vi "compress to 8 bit imaq cast.vi"(8 "error in (no error)":errorcluster, 9 "Image Dst Out":T1, 10 "Bit depth":string, 11 "Refnum in":T1) -> (0 "error out":errorcluster, 3 "Refnum out":T1)   [LabVIEW 2020]
uses:
  IMAQ Image.ctl
  NI_Vision_Development_Module.lvlib
panel:
  in  "lose lowest bits":bool
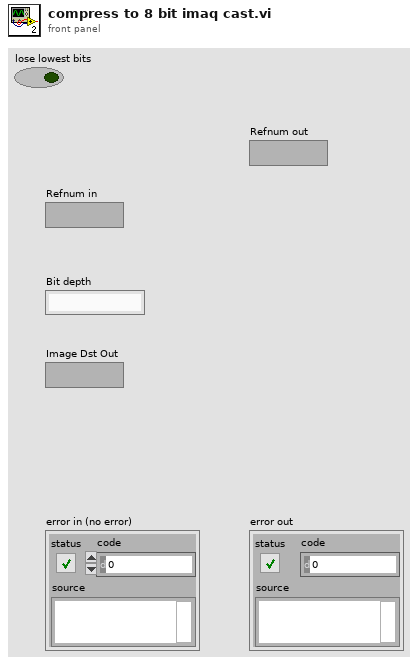
[diagram p1: front panel]
types:
  T1 = typedef "IMAQ Image.ctl" = refnum<image>
  T2 = typedef "Image Type" = u32
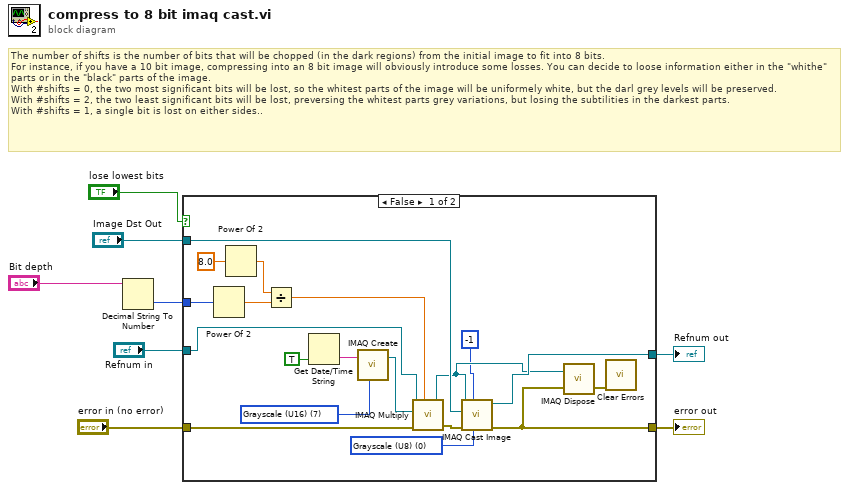
[diagram p0: block diagram]
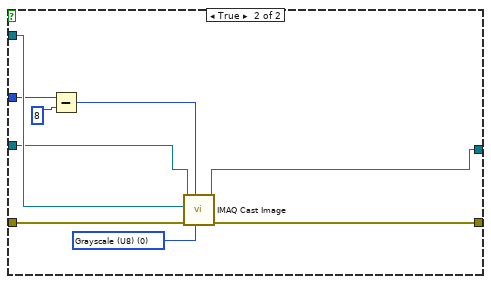
[diagram p2: hidden frame]
diagram:
  # "The number of shifts is the number of bits that will be chopped (in the dark regions) from the initial image to fit into 8 bits.\nFor instance, if you have a 10 bit image, compressing into an 8 bit image will obviously introduce some losses. You can decide to loose information either in the \"whithe\" parts or in the \"black\" parts of the image.\nWith #shifts = 0, the two most significant bits will be lost, so the whitest parts of the image will be uniformely white, but the darl grey levels will be preserved.\nWith #shifts = 2, the two least significant bits will be lost, preversing the whitest parts grey variations, but losing the subtilities in the darkest parts.\nWith #shifts = 1, a single bit is lost on either sides.."
  n1 = Decimal String To Number(string="Bit depth") -> (number=w5:i32)  [unwired: 2 in, 1 out]
  n2 = case shown="False" "lose lowest bits" {
    tunnel: "Image Dst Out" -> [w15 w36]
    tunnel: [w14 w35] -> w7
    tunnel: "error in (no error)" -> [w19 w34]
    tunnel: w5 -> [w25 w32]
    tunnel: [w26 w30] -> w3
    tunnel: "Refnum in" -> [w20 w29]
    frame False {
      w12 = T2 7 items=["Grayscale (U8)", "Grayscale (I16)", "Grayscale (SGL)", "Complex (CSG)", "RGB (U32)", "HSL (U32)", "RGB (U64)", "Grayscale (U16)"] ("Image Type")
      w27 = T2 0 items=["Grayscale (U8)", "Grayscale (I16)", "Grayscale (SGL)", "Complex (CSG)", "RGB (U32)", "HSL (U32)", "RGB (U64)", "Grayscale (U16)"] ("Image Type")
      n3 = Power Of 2(x=w25) -> (2^x=w22:dbl)
      n4 = Power Of 2(x=8.0) -> (2^x=w23:dbl)
      n5 = Divide(x=w23, y=w22) -> (x/y=w21:dbl)
      n6 = Get Date/Time String(want seconds? (F)=TRUE) -> (time string=w17:string)  [unwired: 2 in, 1 out]
      n7 = call "IMAQ Create"("Image Name"=w17, "Image Type"=w12) -> ("New Image"=w16:T1)  [unwired: 3 in, 1 out]
      n8 = call "IMAQ Multiply"("Image Src A"=w20, "Constant"=w21, "Image Dst"=w16, "error in (no error)"=w19) -> ("Image Dst Out"=w13:T1, "error out"=w18:errorcluster)  [unwired: 3 in]
      n9 = call "IMAQ Cast Image"("Image Type"=w27, "# Shifts"=-1, "error in (no error)"=w18, "Image Dst"=w15, "Image Src"=w13) -> ("error out"=w14:errorcluster, "Image Dst Out"=w26:T1)  [unwired: 5 in]
      n10 = call "IMAQ Dispose"("Image"=w13, "error in (no error)"=w14) -> ("error out"=w11:errorcluster)  [unwired: 4 in]
      n11 = call "Clear Errors.vi"("error in (no error)"=w11) -> ()  [unwired: 5 in, 2 out]
    }
    frame True {
      w31 = T2 0 items=["Grayscale (U8)", "Grayscale (I16)", "Grayscale (SGL)", "Complex (CSG)", "RGB (U32)", "HSL (U32)", "RGB (U64)", "Grayscale (U16)"] ("Image Type")
      n12 = Subtract(x=w32, y=8 ("# Shifts")) -> (x-y=w33:i32)
      n13 = call "IMAQ Cast Image"("Image Type"=w31, "# Shifts"=w33, "error in (no error)"=w34, "Image Dst"=w36, "Image Src"=w29) -> ("error out"=w35:errorcluster, "Image Dst Out"=w30:T1)  [unwired: 5 in]
    }
  }
  "error out" <- w7
  "Refnum out" <- w3
